vi "初始化.vi"(8 "error in (no error)":errorcluster caption="错误输入（无错误）", 11 "控制盒（队列） 输入":refnum<class "控制盒（队列）.lvclass"> caption="DNL_LabVIEW Object in") -> (0 "error out":errorcluster caption="错误输出", 3 "控制盒（队列） 输出":refnum<class "控制盒（队列）.lvclass"> caption="DNL_LabVIEW Object out")   [LabVIEW 2011, in "控制盒（队列）.lvclass"]
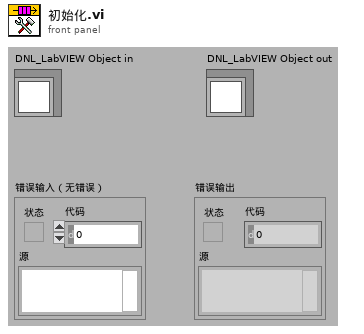
[diagram p1: front panel]
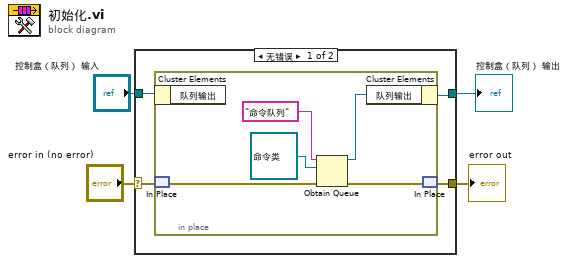
[diagram p0: block diagram]
diagram:
  n1 = case shown="无错误" "error in (no error)" {
    selector: "error in (no error)" -> [w7 w15]
    tunnel: [w6 w15] -> w3
    tunnel: [w5 w14] -> w1
    tunnel: "控制盒（队列） 输入" -> [w8 w14]
    frame No Error {
      n2 = in-place {
        n3 = in-place-cluster #1(w8) -> ()  [unwired: 1 out]
        n4 = in-place-match #2(w7) -> (w12:errorcluster)
        n5 = Obtain Queue(name (unnamed)="命令队列" ("名称（未命名）"), element data type=refnum<class "命令类.lvclass"> refnum ("命令类.lvclass"), error in (no error)=w12) -> (queue out=w9:refnum<queue>, error out=w11:errorcluster)  [unwired: 2 in, 1 out]
        n6 = in-place-cluster #1("队列输出"=w9) -> (w5:refnum<class "控制盒（队列）.lvclass">)
        n7 = in-place-match #2(w11) -> (w6:errorcluster)
      }
    }
    frame Error {
    }
  }
  "error out" <- w3
  "控制盒（队列） 输出" <- w1
